vi "PathPlanning.vi"(0 "Map & Nodes":T2, 1 "error in (no error)":errorcluster) -> (2 "Path":i32[](array[numeric]), 3 "Coordinates":cluster{"X":dbl, "Y":dbl}[](array[cluster]), 4 "error out":errorcluster)   [LabVIEW 2009]
uses:
  <vilib>/Analysis/Matrix/Datatypes/RealMatrix.ctl
  <vilib>/Analysis/Matrix/NI_Matrix.lvlib
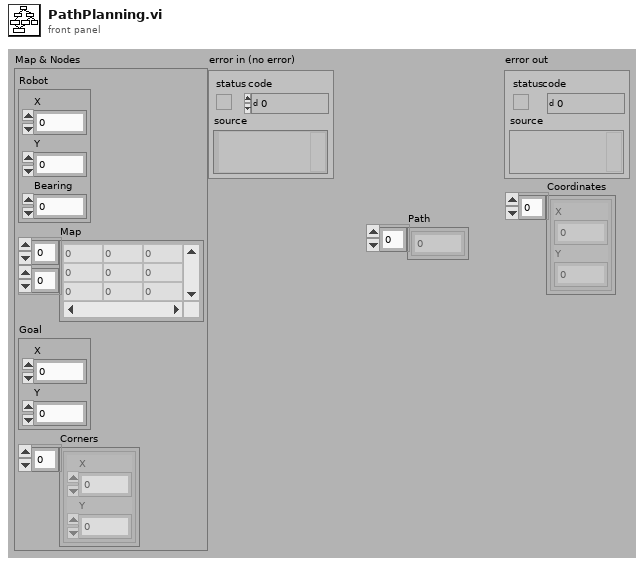
[diagram p1: front panel]
types:
  T1 = typedef "NI_Matrix.lvlib/RealMatrix.ctl" = dbl[][]
  T2 = cluster{"Robot":cluster{"X":dbl, "Y":dbl, "Bearing":dbl}, "Map":T1, "Goal":cluster{"X":dbl, "Y":dbl}, "Corners":cluster{"X":dbl, "Y":dbl}[]}
  T3 = cluster{"From node":cluster{"X":dbl, "Y":dbl}, "Dest node":cluster{"X":dbl, "Y":dbl}, "Distance":dbl, "Dest node no":i32, "From node no":i32}[]
  T4 = cluster{"From node":cluster{"X":dbl, "Y":dbl}, "Dest node":cluster{"X":dbl, "Y":dbl}, "Distance":dbl, "Dest node no":i32, "From node no":i32}
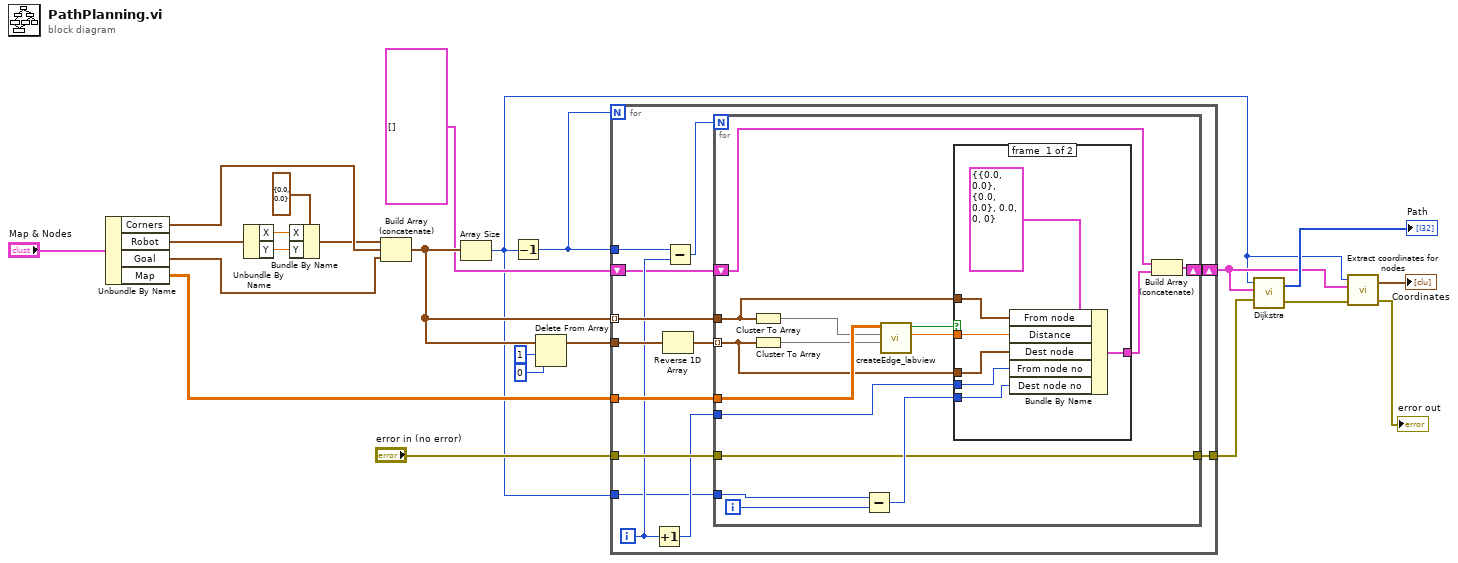
[diagram p0: block diagram]
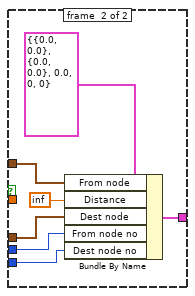
[diagram p2: hidden frame]
diagram:
  n1 = Unbundle By Name("Map & Nodes") -> ("Corners"=w14:cluster{"X":dbl, "Y":dbl}[], "Robot"=w18:cluster{"X":dbl, "Y":dbl, "Bearing":dbl}, "Goal"=w13:cluster{"X":dbl, "Y":dbl}, "Map"=w19:T1)
  n2 = Unbundle By Name(w18) -> ("X"=w17:dbl, "Y"=w16:dbl)
  n3 = Bundle By Name(cluster=cluster{"X":dbl, "Y":dbl} {"X"=0.0, "Y"=0.0} ("Robot 2"), "X"=w17, "Y"=w16) -> (w12:cluster{"X":dbl, "Y":dbl})
  n4 = Build Array (concatenate)(w12, w14, w13) -> (w11:cluster{"X":dbl, "Y":dbl}[])
  n5 = Array Size(array=w11) -> (size(s)=w1:i32)
  n6 = Decrement(x=w1) -> (x-1=w4:i32)
  n7 = Delete From Array(array=w11, length=1, index=0) -> (array with subset deleted=w20:cluster{"X":dbl, "Y":dbl}[])  [unwired: 1 out]
  n8 = for {
    N: w4 -> [_]
    tunnel: w11 -> [w35] mode=indexing
    tunnel: w20 -> [w36]
    tunnel: w19 -> [w34]
    tunnel: w4 -> [w32]
    tunnel: "error in (no error)" -> [w30]
    tunnel: [w29] -> w9
    shift-right: [w33] -> w3
    shift-left: T3 [] -> [w25]
    tunnel: w1 -> [w24]
    i -> [w28]
    n9 = Increment(x=w28) -> (x+1=w27:i32)
    n10 = Reverse 1D Array(array=w36) -> (reversed array=w26:cluster{"X":dbl, "Y":dbl}[])
    n11 = Subtract(x=w32, y=w28) -> (x-y=w31:i32)
    n12 = for {
      N: w31 -> [_]
      tunnel: w26 -> [w47] mode=indexing
      tunnel: w35 -> [w45]
      tunnel: w34 -> [w51]
      tunnel: w27 -> [w43]
      tunnel: w30 -> [w37]
      tunnel: [w37] -> w29
      shift-right: [w42] -> w33
      shift-left: w25 -> [w40]
      tunnel: w24 -> [w38]
      i -> [w39]
      n13 = Cluster To Array(cluster=w45) -> (array=w49:dbl[])
      n14 = Cluster To Array(cluster=w47) -> (array=w48:dbl[])
      n15 = Subtract(x=w38, y=w39) -> (x-y=w44:i32)
      n16 = call "createEdge_labview.vi"("node 2"=w48, "node1"=w49, "Map"=w51) -> ("Distance No COMPLEX"=w46:dbl, "FreePath"=w50:bool)  [unwired: 7 in]
      n17 = case shown="True" w50 {
        tunnel: w47 -> [w54 w62]
        tunnel: w46 -> [w57 _]
        tunnel: w45 -> [w58 w65]
        tunnel: [w55 w63] -> w41
        tunnel: w43 -> [w53 w61]
        tunnel: w44 -> [w52 w60]
        frame #0 {
          n18 = Bundle By Name(cluster=T4 {"From node"={"X"=0.0, "Y"=0.0}, "Dest node"={"X"=0.0, "Y"=0.0}, "Distance"=0.0, "Dest node no"=0, "From node no"=0}, "From node"=w58, "Distance"=w57, "Dest node"=w54, "From node no"=w53, "Dest node no"=w52) -> (w55:T4)
        }
        frame #1 {
          n19 = Bundle By Name(cluster=T4 {"From node"={"X"=0.0, "Y"=0.0}, "Dest node"={"X"=0.0, "Y"=0.0}, "Distance"=0.0, "Dest node no"=0, "From node no"=0}, "From node"=w65, "Distance"=inf, "Dest node"=w62, "From node no"=w61, "Dest node no"=w60) -> (w63:T4)
        }
      }
      n20 = Build Array (concatenate)(w40, w41) -> (w42:T3)
    }
  }
  n21 = call "Dijkstra.vi"("error in (no error)"=w9, "Edges"=w3, "Number of Nodes"=w1) -> ("error out"=w6:errorcluster, "Path"=→"Path":i32[])  [unwired: 1 in]
  n22 = call "Extract coordinates for nodes.vi"("error in (no error)"=w6, "Edges"=w3, "Number of Nodes"=w1) -> ("error out"=→"error out":errorcluster, "Coordinates"=→"Coordinates":cluster{"X":dbl, "Y":dbl}[])  [unwired: 1 in]
